vi "LoadWaveForm.vi"(4 "modulation frequency (Hz)":dbl=32467.5, 9 "Npoint":dbl=1000.0, 10 "arbitrary parameters":T1={"max number of waveforms"=4, "waveform quantum"=1, "max waveform size"=131072, "min waveform size"=2}) -> (1 "waveform":dbl[](array[numeric]))   [LabVIEW 2015, in "ArbitraryFunctions.lvlib"]
uses:
  ArbitraryFunctions.lvlib
  <vilib>/Analysis/baseanly.llb/Mean (DBL).vi
  <vilib>/Analysis/NI_AALBase.lvlib
panel:
  in  "Tab Control 2":enum32{"function screens", "configuration"}(tab)
  out "frequency profile":cluster{dbl[], "Windowed X":dbl[]}(graph)
  in  "X axis":enum16{"time(ms)", "time(us)", "points"}(ring)
  out "temporal profile":cluster{dbl[], dbl[]}(graph)
  out "dt (s)":dbl
  in  "Tab Control":T2(tab)
  in  "gaussian parameters":cluster{"n":i16, "delay":i32, "sigma":i32}={"n"=2, "delay"=10, "sigma"=10} {"sigma" min=1}
  in  "Low Frequency":dbl=100000.0
  in  "High Frequency IN":dbl=80000000.0
  in  "Nrep Low":dbl
  in  "Phase (2pi unit)":dbl=80000000.0
  in  "Nrep":dbl
  in  "N point":i32=1000
  in  "delay":i32=100
  in  "length":i32=100
  in  "number of phases":i32=4 min=1
  in  "Nz":dbl=20.0
  in  "Tau_expo (us)":dbl=1e-06
  in  "chirp":dbl=100000.0 min=1.0
  in  "N rep":dbl=20.0
  in  "Npoints":i32
  in  "Phase (2pi unit)":dbl=80000000.0
  in  "OK Button":bool
  # "Npoints = 1000 for PM modulation\nto work\n\nNpoint can be increased to maximum when \narbitrary waveform is generated"
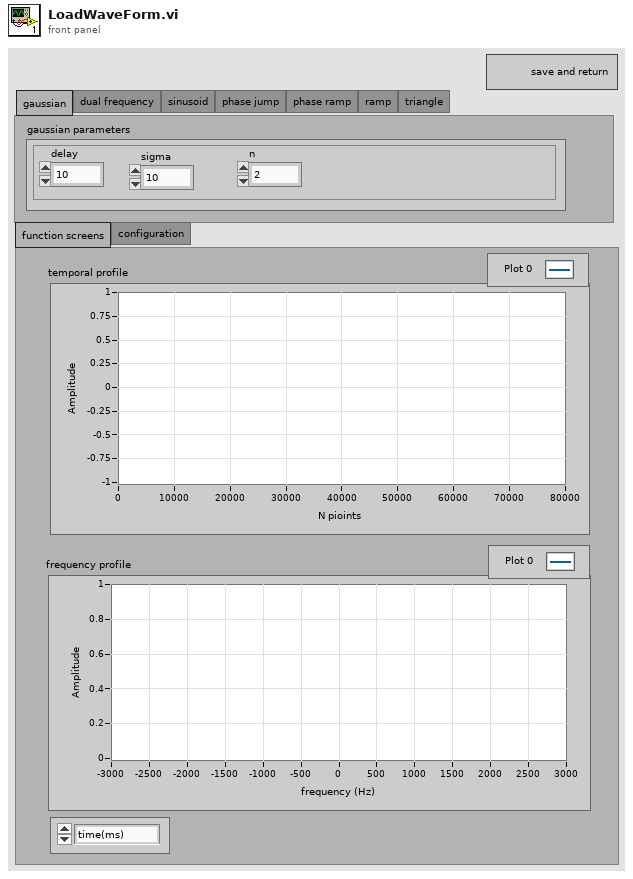
[diagram p1: front panel]
types:
  T1 = cluster{"max number of waveforms":i32, "waveform quantum":i32, "max waveform size":i32, "min waveform size":i32}
  T2 = enum32{"gaussian", "dual frequency", "sinusoid", "phase jump", "phase ramp", "ramp", "triangle"}
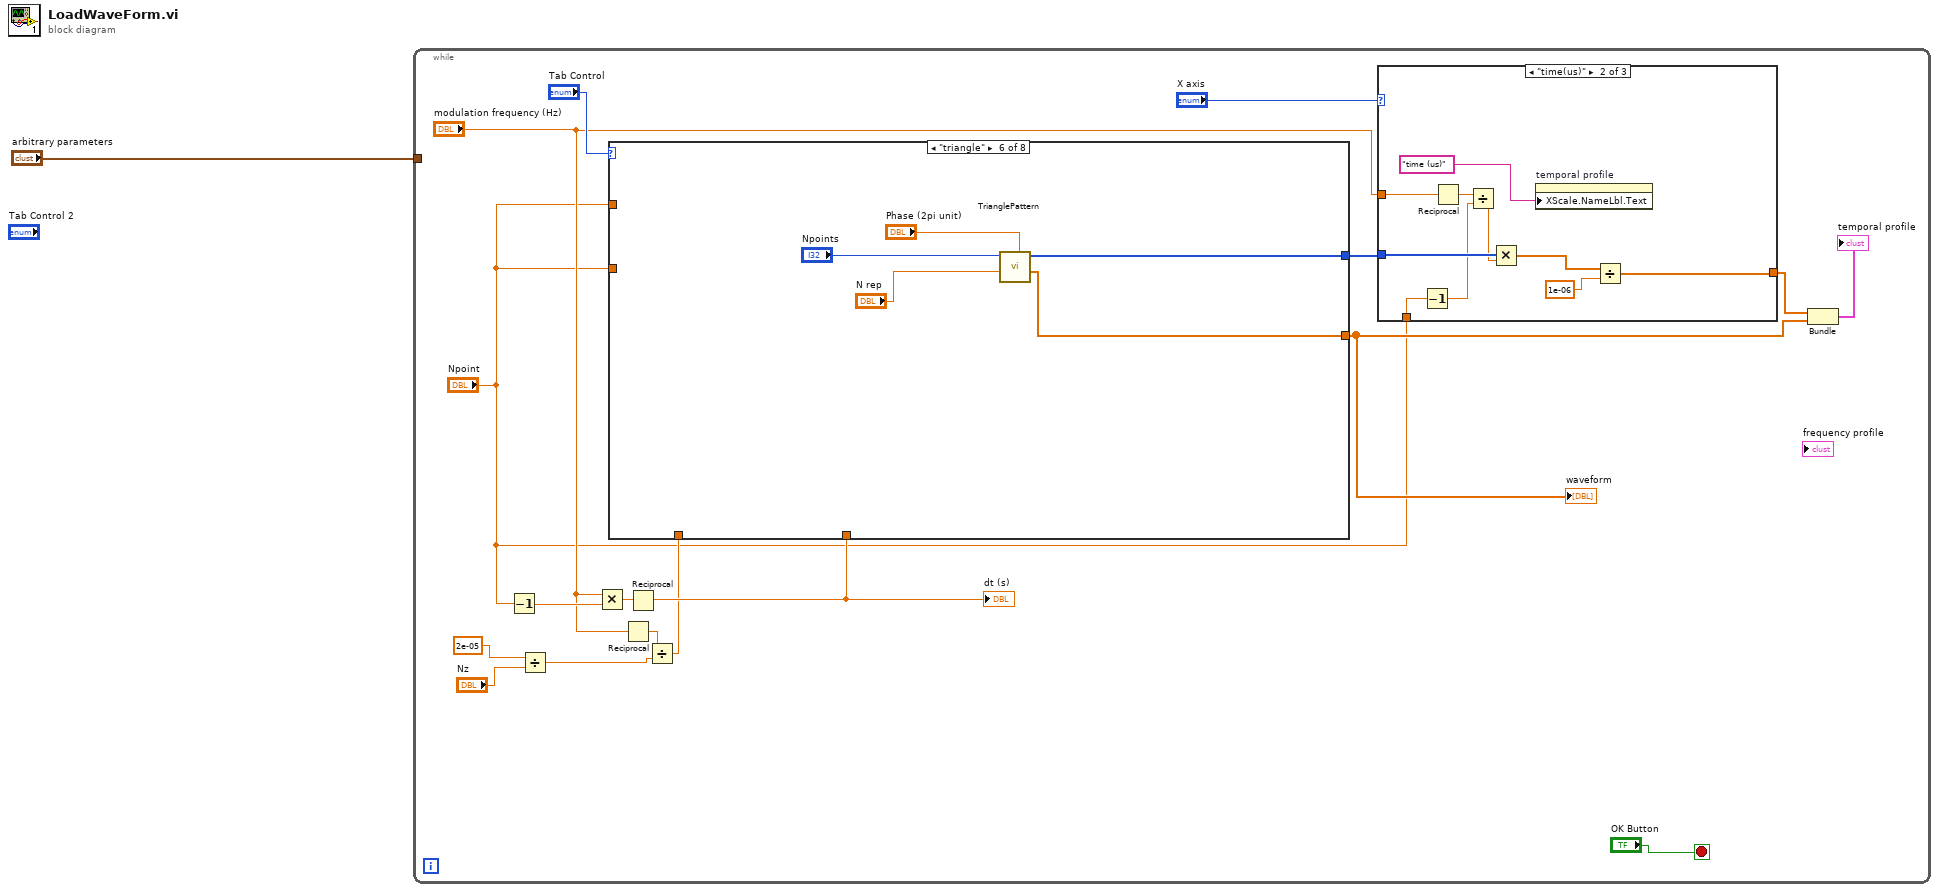
[diagram p0: block diagram]
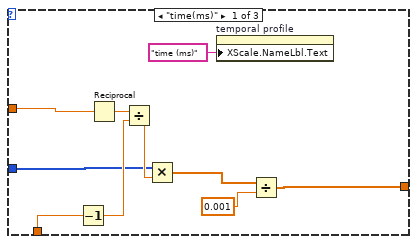
[diagram p2: hidden frame]
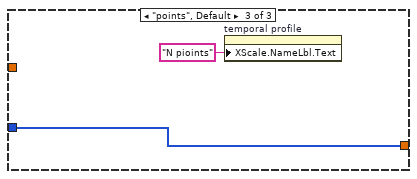
[diagram p3: hidden frame]
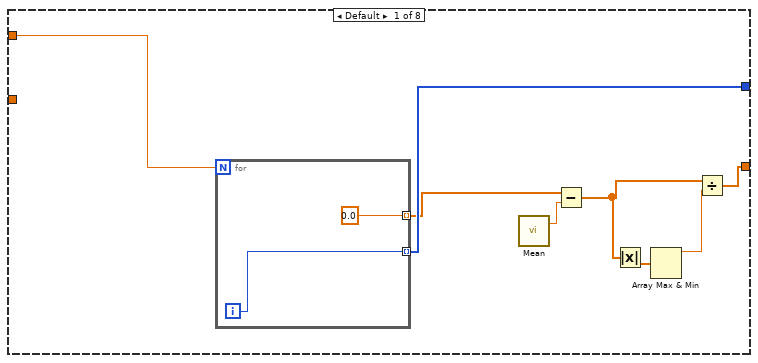
[diagram p4: hidden frame]
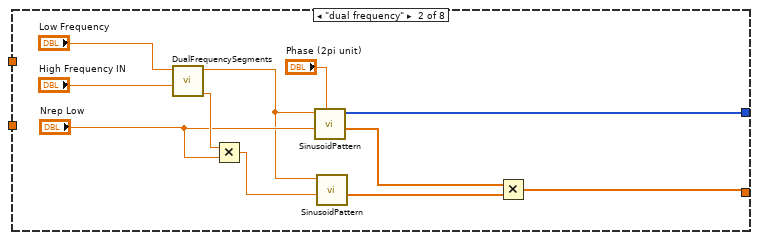
[diagram p5: hidden frame]
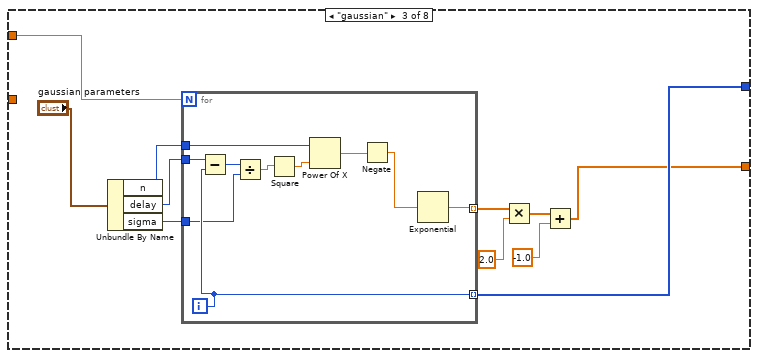
[diagram p6: hidden frame]
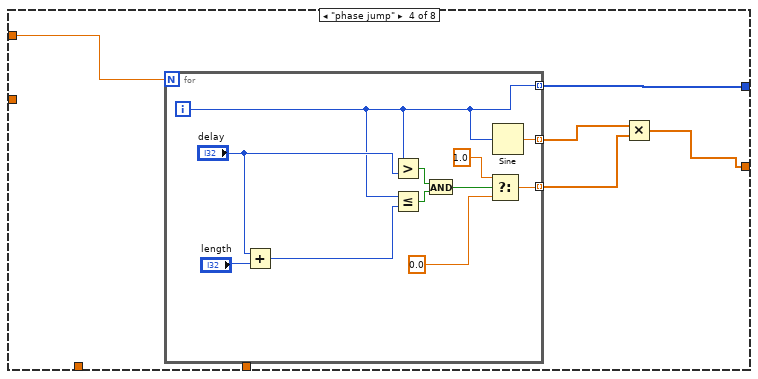
[diagram p7: hidden frame]
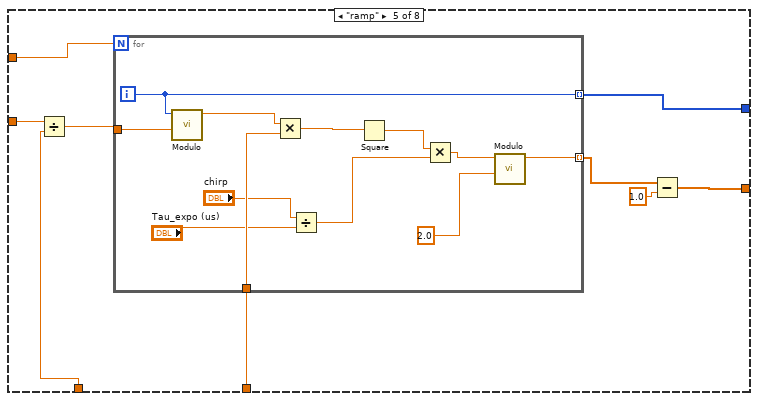
[diagram p8: hidden frame]
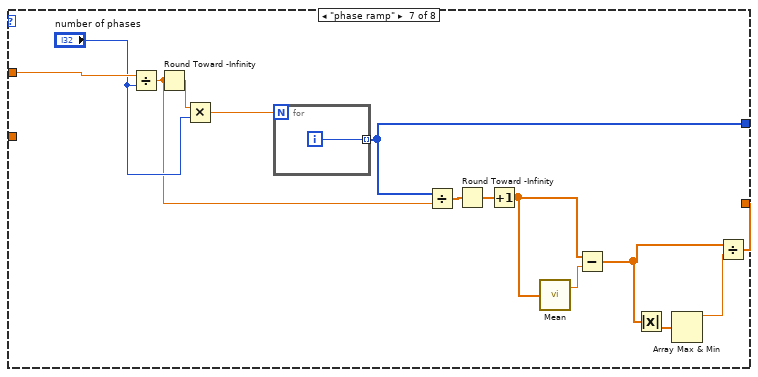
[diagram p9: hidden frame]
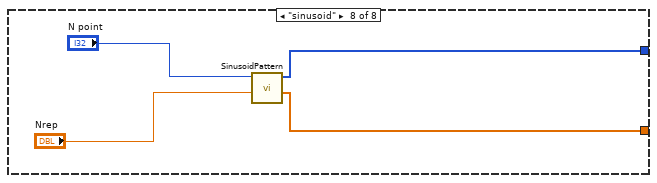
[diagram p10: hidden frame]
diagram:
  n1 = while {
    tunnel: "arbitrary parameters" -> [_]
    stop <- "OK Button" stop-if-true
    n2 = Decrement(x="Npoint") -> (x-1=w11:dbl)
    n3 = Divide(x=2e-05, y="Nz") -> (x/y=w4:dbl)
    n4 = Multiply(x="modulation frequency (Hz)", y=w11) -> (x*y=w8:dbl)
    n5 = Reciprocal(x="modulation frequency (Hz)") -> (1/x=w5:dbl)
    n6 = Reciprocal(x=w8) -> (1/x=w7:dbl)
    "dt (s)" <- w7
    n7 = Divide(x=w5, y=w4) -> (x/y=w3:dbl)
    n8 = case shown="\"triangle\"" "Tab Control" {
      tunnel: "Npoint" -> [w47 _ w72 w87 w102 _ w138 _]
      tunnel: [w48 w59 w71 w86 w105 w124 w135 w141] -> w12
      tunnel: [w41 w53 w64 w83 w103 w123 w125 w142] -> w16
      tunnel: w7 -> [_ _ _ _ w107 _ _ _]
      tunnel: w3 -> [_ _ _ _ w101 _ _ _]
      tunnel: "Npoint" -> [_ _ _ _ w100 _ _ _]
      frame Default {
        n9 = for {
          N: w47 -> [_]
          tunnel: [w50] -> w48 mode=indexing
          tunnel: [0.0] -> w42 mode=indexing
          i -> [w50]
        }
        n10 = call-poly <vilib>:"Mean.vi"() -> ("mean"=w44:dbl)  [unwired: 1 in, 1 out]
        n11 = Subtract(x=w42, y=w44) -> (x-y=w45:dbl[])
        n12 = Absolute Value(x=w45) -> (abs(x)=w46:dbl[])
        n13 = Array Max & Min(array=w46) -> (max value=w43:dbl)  [unwired: 3 out]
        n14 = Divide(x=w45, y=w43) -> (x/y=w41:dbl[])
      }
      frame "dual frequency" {
        n15 = call "DualFrequencySegments.vi"("High Frequency IN"="High Frequency IN", "Low Frequency"="Low Frequency") -> ("N high - low"=w58:dbl, "N points"=w56:dbl)  [unwired: 7 in, 1 out]
        n16 = Multiply(x=w58, y="Nrep Low") -> (x*y=w55:dbl)
        n17 = call "SinusoidPattern.vi"("Phase (2pi unit)"="Phase (2pi unit)", "Nrep"="Nrep Low", "N point"=w56) -> ("Unit Pattern"=w54:dbl[], "Points"=w59:i32[])  [unwired: 7 in]
        n18 = call "SinusoidPattern.vi"("Nrep"=w55, "N point"=w56) -> ("Unit Pattern"=w52:dbl[])  [unwired: 8 in, 1 out]
        n19 = Multiply(x=w54, y=w52) -> (x*y=w53:dbl[])
      }
      frame "gaussian" {
        n20 = Unbundle By Name("gaussian parameters") -> ("n"=w69:i16, "delay"=w68:i32, "sigma"=w67:i32)
        n21 = for {
          N: w72 -> [_]
          tunnel: [w82] -> w71 mode=indexing
          tunnel: [w81] -> w65 mode=indexing
          tunnel: w69 -> [w75]
          tunnel: w68 -> [w74]
          tunnel: w67 -> [w73]
          i -> [w82]
          n22 = Subtract(x=w74, y=w82) -> (x-y=w80:i32)
          n23 = Divide(x=w80, y=w73) -> (x/y=w79:dbl)
          n24 = Square(x=w79) -> (x^2=w78:dbl)
          n25 = Power Of X(1:w78, 2:w75) -> (0:w77:dbl)
          n26 = Negate(x=w77) -> (-x=w76:dbl)
          n27 = Exponential(1:w76) -> (0:w81:dbl)
        }
        n28 = Multiply(x=w65, y=2.0) -> (x*y=w62:dbl[])
        n29 = Add(x=w62, y=-1.0) -> (x+y=w64:dbl[])
      }
      frame "phase jump" {
        n30 = for {
          N: w87 -> [_]
          tunnel: [w89] -> w86 mode=indexing
          tunnel: [w93] -> w84 mode=indexing
          tunnel: [w88] -> w85 mode=indexing
          i -> [w89]
          n31 = Add(x="delay", y="length") -> (x+y=w90:i32)
          n32 = Greater?(x=w89, y="delay") -> (0:w97:bool)
          n33 = Less Or Equal?(x=w89, y=w90) -> (x <= y?=w96:bool)
          n34 = And(x=w97, y=w96) -> (x .and. y?=w95:bool)
          n35 = Select(t=1.0, s=w95, f=0.0) -> (s? t:f=w93:dbl)
          n36 = Sine(x=w89) -> (sin(x)=w88:dbl)
        }
        n37 = Multiply(x=w85, y=w84) -> (x*y=w83:dbl[])
      }
      frame "ramp" {
        n38 = Divide(x=w100, y=w101) -> (x/y=w99:dbl)
        n39 = for {
          N: w102 -> [_]
          tunnel: [w116] -> w105 mode=indexing
          tunnel: [w115] -> w104 mode=indexing
          tunnel: w107 -> [w119]
          tunnel: w99 -> [w114]
          i -> [w116]
          n40 = call "Modulo.vi"("mod"=w114, "input"=w116) -> ("output"=w113:dbl)  [unwired: 9 in]
          n41 = Multiply(x=w113, y=w119) -> (x*y=w118:dbl)
          n42 = Divide(x="chirp", y="Tau_expo (us)") -> (x/y=w110:dbl)
          n43 = Square(x=w118) -> (x^2=w111:dbl)
          n44 = Multiply(x=w111, y=w110) -> (x*y=w109:dbl)
          n45 = call "Modulo.vi"("mod"=2.0 ("y"), "input"=w109) -> ("output"=w115:dbl)  [unwired: 9 in]
        }
        n46 = Subtract(x=w104, y=1.0) -> (x-y=w103:dbl[])
      }
      frame "triangle" {
        n47 = call "TrianglePattern.vi"("Phase (2pi unit)"="Phase (2pi unit)", "N rep"="N rep", "N"="Npoints") -> ("vector"=w123:dbl[], "points"=w124:i32[])  [unwired: 7 in]
      }
      frame "phase ramp" {
        n48 = Divide(x=w138, y="number of phases") -> (x/y=w133:dbl)
        n49 = Round Toward -Infinity(1:w133) -> (0:w136:dbl)
        n50 = Multiply(x=w136, y="number of phases") -> (x*y=w137:dbl)
        n51 = for {
          N: w137 -> [_]
          tunnel: [w139] -> w135 mode=indexing
          i -> [w139]
        }
        n52 = Divide(x=w135, y=w133) -> (x/y=w132:dbl[])
        n53 = Round Toward -Infinity(1:w132) -> (0:w131:dbl[])
        n54 = Increment(x=w131) -> (x+1=w126:dbl[])
        n55 = call-poly <vilib>:"Mean.vi"("X"=w126) -> ("mean"=w128:dbl)  [unwired: 1 out]
        n56 = Subtract(x=w126, y=w128) -> (x-y=w129:dbl[])
        n57 = Absolute Value(x=w129) -> (abs(x)=w130:dbl[])
        n58 = Array Max & Min(array=w130) -> (max value=w127:dbl)  [unwired: 3 out]
        n59 = Divide(x=w129, y=w127) -> (x/y=w125:dbl[])
      }
      frame "sinusoid" {
        n60 = call "SinusoidPattern.vi"("Nrep"="Nrep", "N point"="N point") -> ("Unit Pattern"=w142:dbl[], "Points"=w141:i32[])  [unwired: 8 in]
      }
    }
    "waveform" <- w16
    n61 = case shown="\"time(us)\"" "X axis" {
      tunnel: [w20 w31 w40] -> w13
      tunnel: w12 -> [w21 w38 w40]
      tunnel: "Npoint" -> [w23 w36 _]
      tunnel: "modulation frequency (Hz)" -> [w22 w30 _]
      frame "time(ms)" {
        n62 = Decrement(x=w23) -> (x-1=w27:dbl)
        n63 = Reciprocal(x=w22) -> (1/x=w28:dbl)
        n64 = Divide(x=w28, y=w27) -> (x/y=w26:dbl)
        n65 = Multiply(x=w21, y=w26) -> (x*y=w24:dbl[])
        n66 = property on="temporal profile" class="XYGraph (strict)"("XScale.NameLbl.Text"="time (ms)" ("X Scale.Name Label.Text")) -> ()  [unwired: 2 in, 2 out]
        n67 = Divide(x=w24, y=0.001) -> (x/y=w20:dbl[])
      }
      frame "time(us)" {
        n68 = Decrement(x=w36) -> (x-1=w35:dbl)
        n69 = Reciprocal(x=w30) -> (1/x=w37:dbl)
        n70 = Divide(x=w37, y=w35) -> (x/y=w34:dbl)
        n71 = Multiply(x=w38, y=w34) -> (x*y=w32:dbl[])
        n72 = property on="temporal profile" class="XYGraph (strict)"("XScale.NameLbl.Text"="time (us)" ("X Scale.Name Label.Text")) -> ()  [unwired: 2 in, 2 out]
        n73 = Divide(x=w32, y=1e-06) -> (x/y=w31:dbl[])
      }
      frame "points", Default {
        n74 = property on="temporal profile" class="XYGraph (strict)"("XScale.NameLbl.Text"="N pioints" ("X Scale.Name Label.Text")) -> ()  [unwired: 2 in, 2 out]
      }
    }
    n75 = Bundle("Points"=w13, "Unit Pattern"=w16) -> (→"temporal profile":cluster{"Points":dbl[], "Unit Pattern":dbl[]})  [unwired: 1 in]
  }
